vi "OpenConnection.vi"(8 "error in":errorcluster, 11 "T560Session in":refnum<class "T560Session.lvclass">) -> (0 "error out":errorcluster, 3 "T560Session out":refnum<class "T560Session.lvclass">)   [LabVIEW 2013, in "T560Session.lvclass"]
doc: "Connect to the T560 physical device"
uses:
  T560Session.lvclass
  T560Session.lvclass/T560Session.ctl
  <vilib>/Instr/_visa.llb/VISA Configure Serial Port (Instr).vi
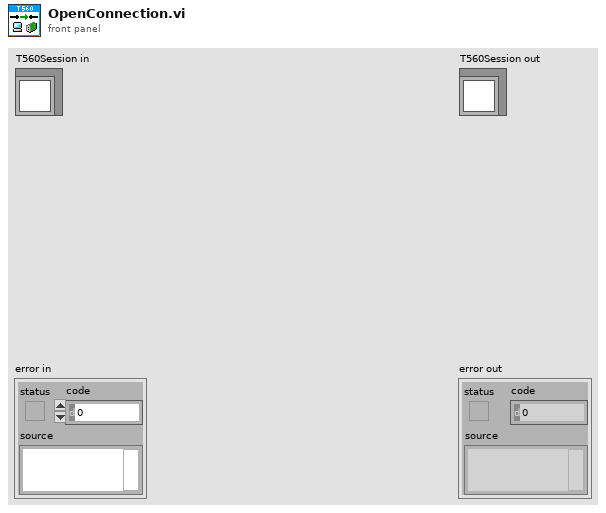
[diagram p1: front panel]
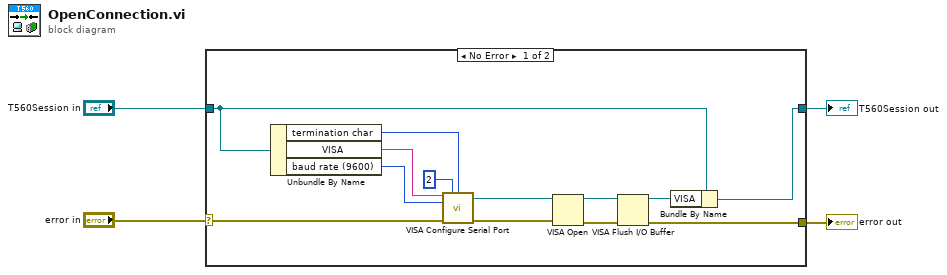
[diagram p0: block diagram]
diagram:
  n1 = case shown="No Error" "error in" {
    selector: "error in" -> [w17 w19]
    tunnel: [w12 w19] -> w3
    tunnel: [w7 w18] -> w1
    tunnel: "T560Session in" -> [w8 w18]
    frame No Error {
      n2 = Unbundle By Name(w8) -> ("termination char"=w9:u8, "VISA"=w11:string, "baud rate (9600)"=w10:u32)
      n3 = call-poly "VISA Configure Serial Port"("VISA resource name"=w11, "timeout (10sec)"=u32 2, "termination char\n(0xA = '\\n' = LF)"=w9, "baud rate (9600)"=w10, "error in (no error)"=w17) -> ("VISA resource name out"=w13:refnum<visa-resource-name>, "error out"=w14:errorcluster)  [unwired: 9 in]
      n4 = VISA Open(error in (no error)=w14, VISA resource name=w13) -> (VISA resource name=w15:refnum<visa-resource-name>, error out=w16:errorcluster)  [unwired: 3 in]
      n5 = VISA Flush I/O Buffer(VISA resource name=w15, error in (no error)=w16) -> (VISA resource name out=w6:refnum<visa-resource-name>, error out=w12:errorcluster)  [unwired: 1 in]
      n6 = Bundle By Name(cluster=w8, "VISA"=w6) -> (w7:refnum<class "T560Session.lvclass">)
    }
    frame Error {
    }
  }
  "error out" <- w3
  "T560Session out" <- w1
